vi "GateGrid.vi"() -> ()   [LabVIEW 2021]
uses:
  <userlib>/Nanonis Prog Interface V5/Nanonis Prog Interface.lvlib
panel:
  in  "milliseconds to wait between grids":u32
  in  "Gate voltages, Start Bias, End Bias (V)":dbl[][](array[numeric])
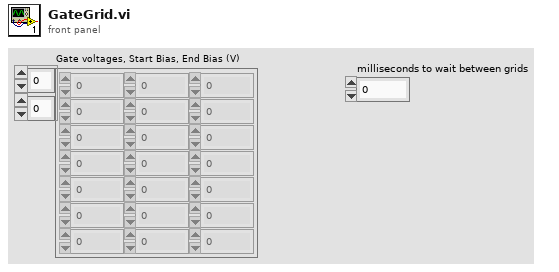
[diagram p1: front panel]
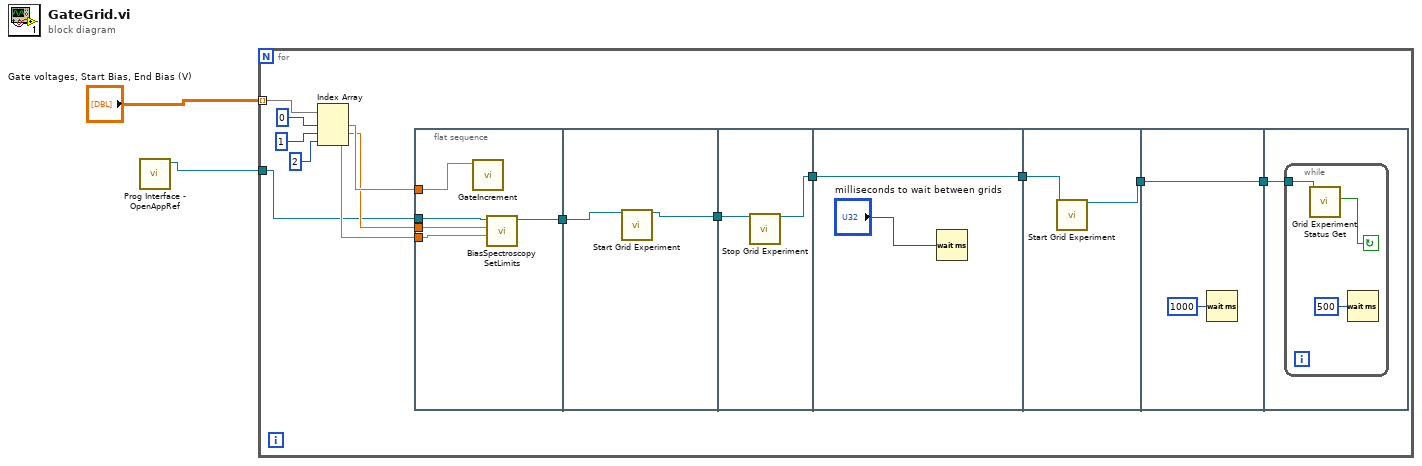
[diagram p0: block diagram]
diagram:
  n1 = call <userlib>:"Prog Interface - OpenAppRef.vi"() -> ("Application reference"=w1:refnum<vi>)  [unwired: 6 in, 1 out]
  n2 = for {
    tunnel: "Gate voltages, Start Bias, End Bias (V)" -> [w16] mode=indexing
    tunnel: w1 -> [w9]
    n3 = Index Array(array=w16, index #1=0 ("index"), index #2=1 ("index"), index #3=2 ("index")) -> (element #1=w12:dbl, element #2=w11:dbl, element #3=w10:dbl)
    n4 = flat-sequence {
      tunnel: w12 -> [w21]
      tunnel: w11 -> [w20]
      tunnel: w10 -> [w19]
      tunnel: w9 -> [w18]
      tunnel: [w17] -> w8
      tunnel: w8 -> [w23]
      tunnel: [w22] -> w7
      tunnel: w7 -> [w25]
      tunnel: [w24] -> w5
      tunnel: [w26] -> w6
      tunnel: w5 -> [w26]
      tunnel: w6 -> [w29]
      tunnel: [w28] -> w4
      tunnel: w4 -> [w31]
      tunnel: [w31] -> w3
      tunnel: w3 -> [w32]
      frame #0 {
        n5 = call "GateIncrement.vi"("Gate Voltage"=w21) -> ()  [unwired: 11 in]
        n6 = call <userlib>:"BiasSpectroscopy SetLimits.vi"("End value (V)"=w19, "Start value (V)"=w20, "Application ref in"=w18) -> ("Application ref out"=w17:refnum<vi>)  [unwired: 5 in, 1 out]
      }
      frame #1 {
        n7 = call <userlib>:"Start Grid Experiment.vi"("Application ref in"=w23) -> ("Application ref out"=w22:refnum<vi>)  [unwired: 17 in, 1 out]
      }
      frame #2 {
        n8 = call <userlib>:"Stop Grid Experiment.vi"("Application ref in"=w25) -> ("Application ref out"=w24:refnum<vi>)  [unwired: 17 in, 1 out]
      }
      frame #3 {
        n9 = Wait (ms)(milliseconds to wait="milliseconds to wait between grids") -> ()  [unwired: 1 out]
      }
      frame #4 {
        n10 = call <userlib>:"Start Grid Experiment.vi"("Application ref in"=w29) -> ("Application ref out"=w28:refnum<vi>)  [unwired: 17 in, 1 out]
      }
      frame #5 {
        n11 = Wait (ms)(milliseconds to wait=u32 1000) -> ()  [unwired: 1 out]
      }
      frame #6 {
        n12 = while {
          tunnel: w32 -> [w34]
          stop <- w35 continue-if-true
          n13 = call <userlib>:"Grid Experiment Status Get.vi"("Application ref in"=w34) -> ("Running?"=w35:bool)  [unwired: 8 in, 2 out]
          n14 = Wait (ms)(milliseconds to wait=u32 500) -> ()  [unwired: 1 out]
        }
      }
    }
  }
